vi "simflight.vi"() -> ()   [LabVIEW 2014]
uses:
  <vilib>/addons/Control Design/_Model Construction/Model Creation.llb/Model Creation SubVI/cd_Create State Space Model.vi
  <vilib>/addons/Control Design/_Utility/Model Viewer.llb/Model Viewer SubVI/cd_Draw State-Space Equation (SS).vi
  <vilib>/Utility/inputDevices.llb/joystickAcquire.vi
  <vilib>/addons/Control Design/_Time Response Analysis/Time Response.llb/Time Response subVI/cd_Linear Simulation (State-Space).vi
  <vilib>/addons/Control Design/_Time Response Analysis/NI_CD_Time Response.lvlib
  <vilib>/addons/Control Design/_Utility/NI_CD_Model Viewer.lvlib
  <vilib>/Analysis/NI_AALPro.lvlib
  <vilib>/Analysis/8numeric.llb/1D Numeric Integration.vi
  <vilib>/addons/Control Design/_Model Construction/NI_LinSys_Model Creation.lvlib
panel:
  out "flight path angle 2":dbl[](graph)
  out "XY Graph 2":cluster{"Y":dbl[], "Y":dbl[]}[](graph)
  out "horsepower":dbl[](graph)
  out "airspeed":dbl[](graph)
  out "elevator command":dbl[](graph)
  out "altitude":dbl[](graph)
  out "flight path angle":dbl[](graph)
  out "pitch rate":dbl[](graph)
  out "Equation 2":picture
  in  "stop":bool
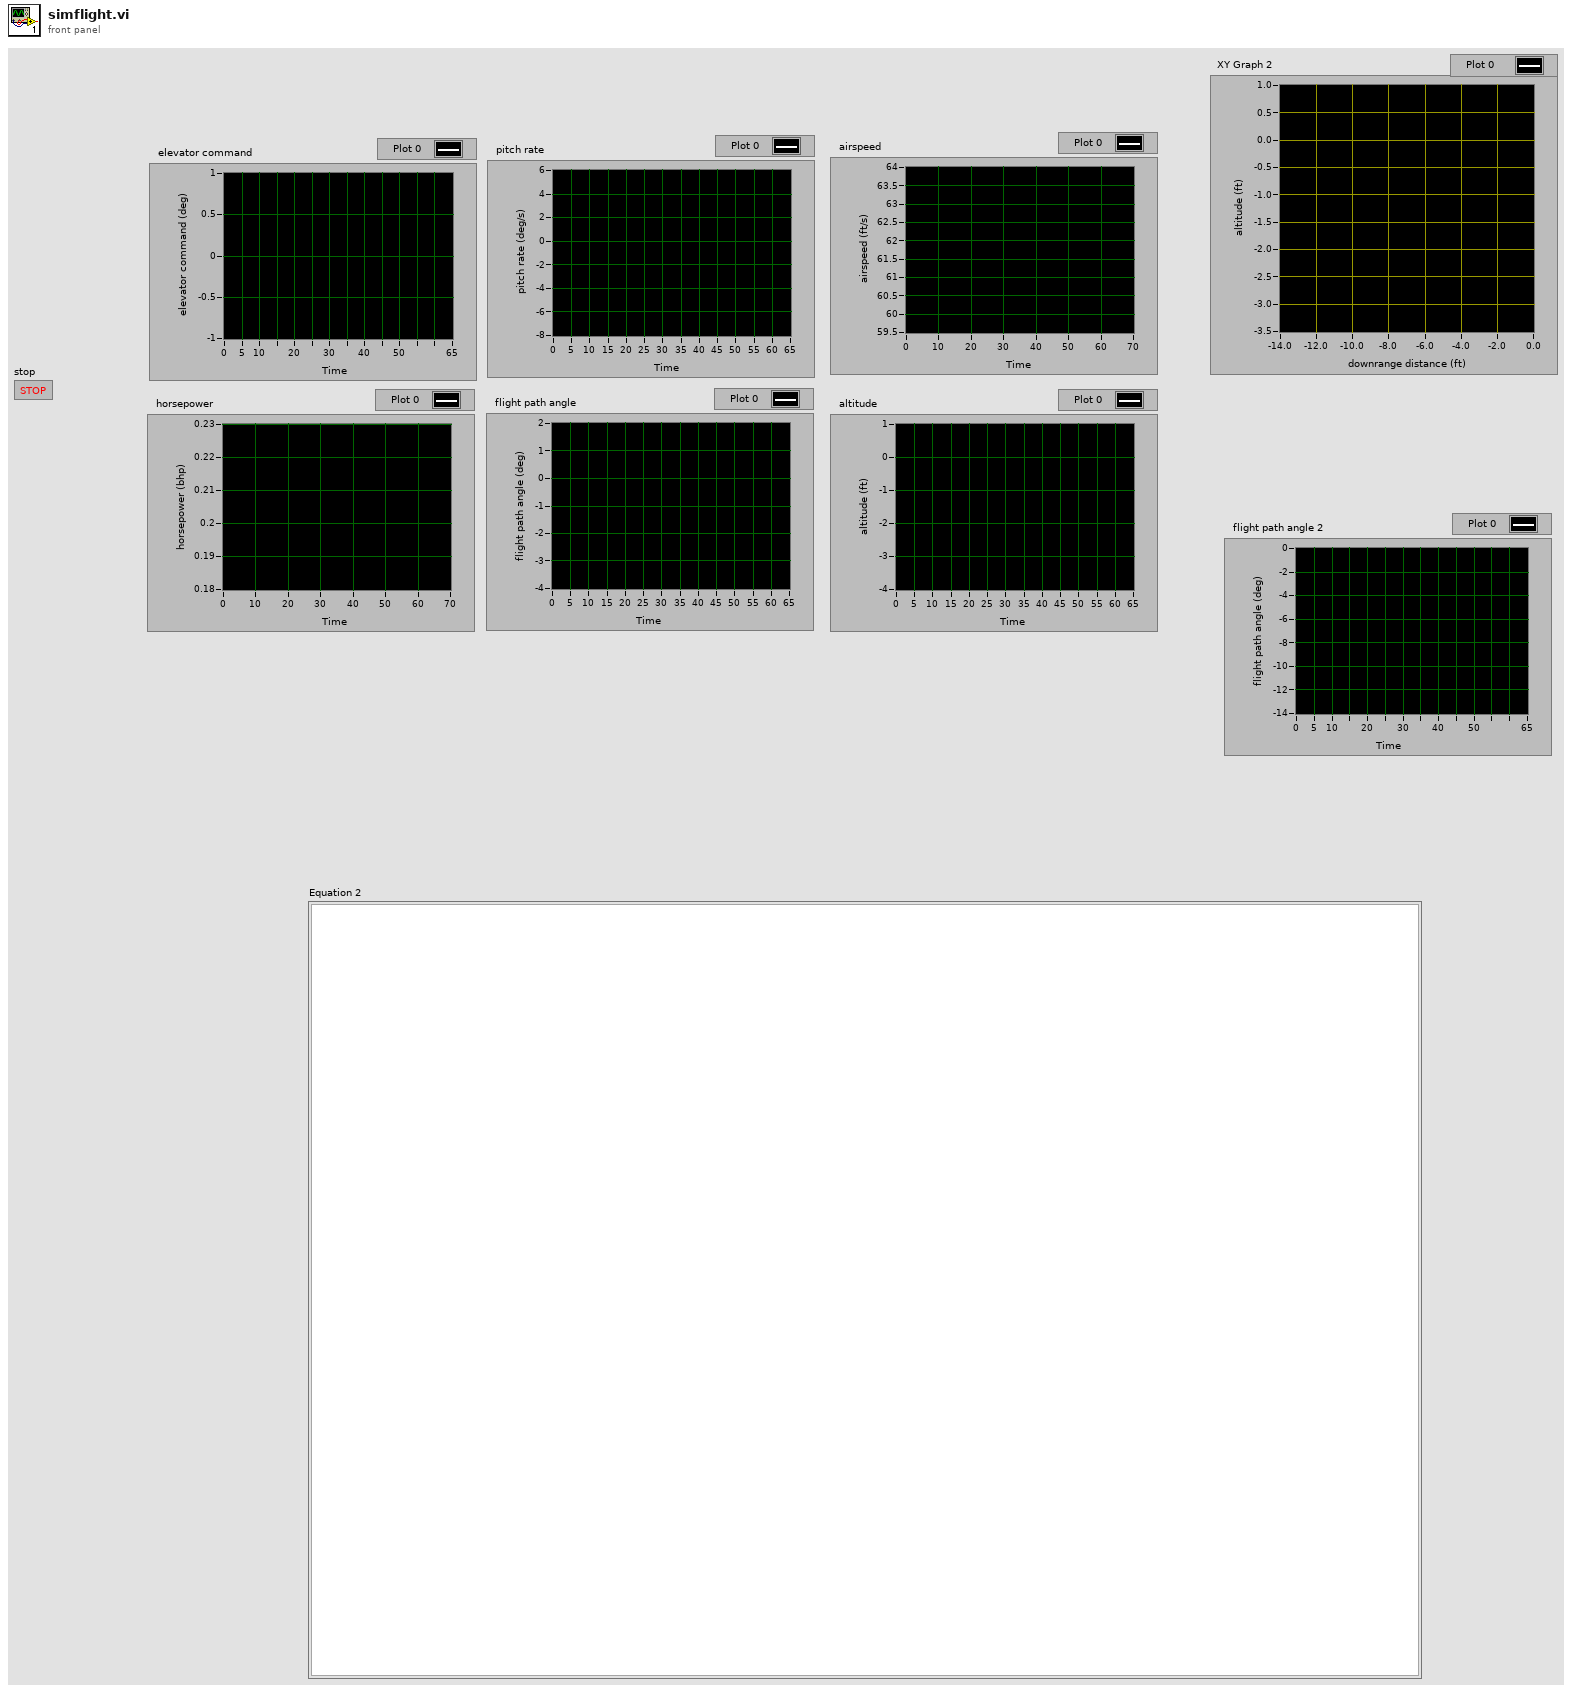
[diagram p1: front panel]
types:
  T1 = typedef "NI_LinSys_Model Typedefs.lvlib/CD State Space Model (MIMO).ctl" = cluster{"properties":T2, "A":dbl[][], "B":dbl[][], "C":dbl[][], "D":dbl[][], "StateNames":string[], "Transport Delay":dbl[][]}
  T2 = typedef "NI_LinSys_Model Typedefs.lvlib/CD General Elements.ctl" = cluster{"Model name":string, "Input names":string[], "Output names":string[], "Input Delays":dbl[], "Output Delays":dbl[], "Sampling Time":dbl, "Notes":string}
  T3 = cluster{"X axis":i32, "Y axis":i32, "Z axis":i32, "X axis rotation":i32, "Y axis rotation":i32, "Z axis rotation":i32, "U axis":i32, "V axis":i32}
  T4 = typedef "NI_LinSys_Data Typedefs.lvlib/CD MIMO Time Response Data.ctl" = cluster{"Time":dbl[], "Outputs Data":dbl[][][], "States Data":dbl[][][], "plot type":T5}
  T5 = typedef "NI_LinSys_Data Typedefs.lvlib/CD Plot Types Enum.ctl" = enum16{"bode-magnitude", "bode-phase", "nichols", "nyquist", "singular values", "step", "impulse", "initial", "simulation", "nyquist with separation"}
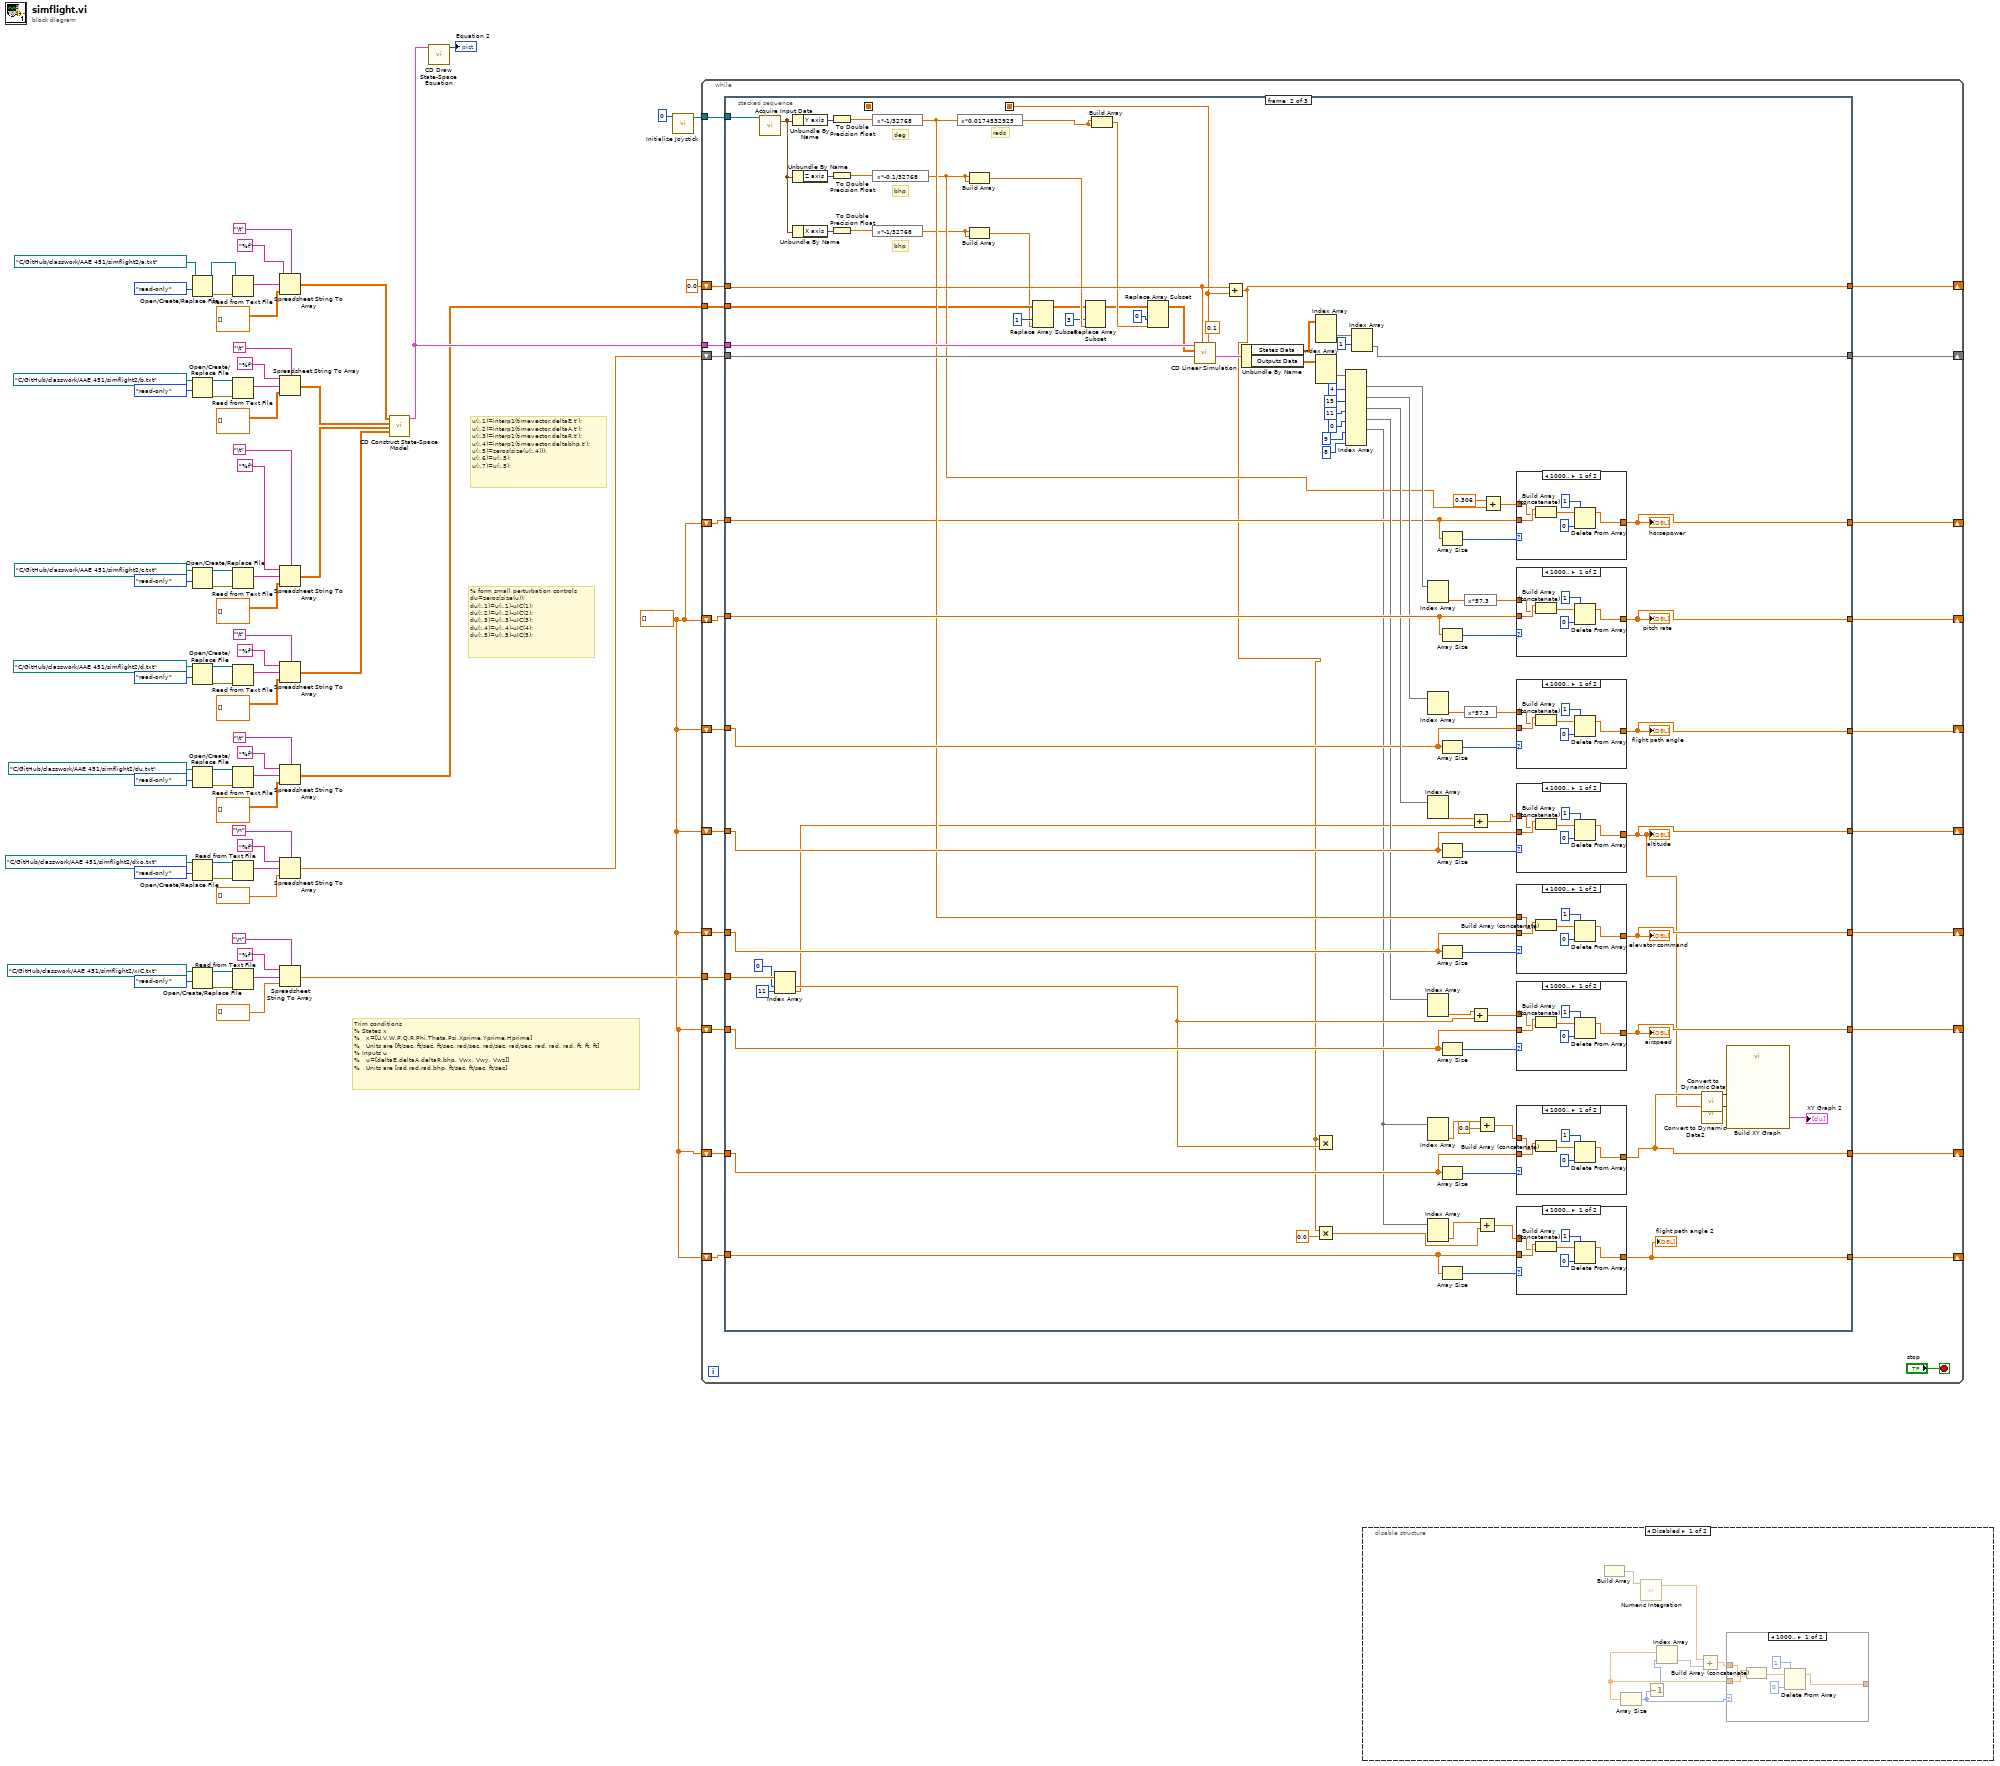
[diagram p0: block diagram]
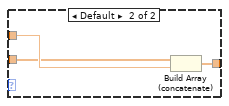
[diagram p2: hidden frame]
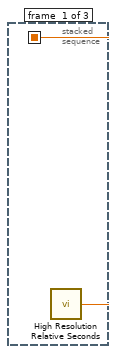
[diagram p4: hidden frame]
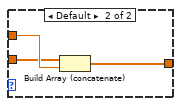
[diagram p5: hidden frame]
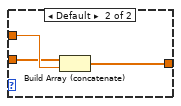
[diagram p6: hidden frame]
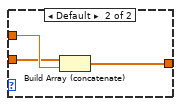
[diagram p7: hidden frame]
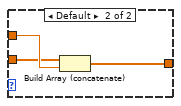
[diagram p8: hidden frame]
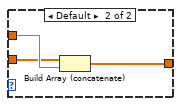
[diagram p9: hidden frame]
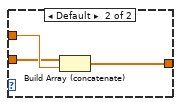
[diagram p10: hidden frame]
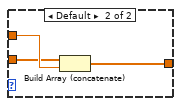
[diagram p11: hidden frame]
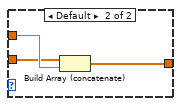
[diagram p12: hidden frame]
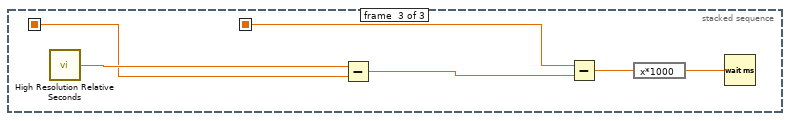
[diagram p13: hidden frame]
diagram:
  w1 = dbl[] []
  # "Trim conditions\n% States x\n%   x=[U,V,W,P,Q,R,Phi,Theta,Psi,Xprime,Yprime,Hprime]\n%   Units are [ft/sec, ft/sec, ft/sec, rad/sec, rad/sec, rad/sec, rad, rad, rad, ft, ft, ft]\n% Inputs u\n%   u=[deltaE,deltaA,deltaR,bhp, Vwx, Vwy, Vwz]]\n%   Units are [rad,rad,rad,bhp, ft/sec, ft/sec, ft/sec]"
  # "% form small perturbation controls\ndu=zeros(size(u));\ndu(:,1)=u(:,1)-uIC(1);\ndu(:,2)=u(:,2)-uIC(2);\ndu(:,3)=u(:,3)-uIC(3);\ndu(:,4)=u(:,4)-uIC(4);\ndu(:,5)=u(:,5)-uIC(5);"
  # "u(:,1)=interp1(timevector,deltaE,t');\nu(:,2)=interp1(timevector,deltaA,t');\nu(:,3)=interp1(timevector,deltaR,t');\nu(:,4)=interp1(timevector,deltabhp,t');\nu(:,5)=zeros(size(u(:,4)));\nu(:,6)=u(:,5);\nu(:,7)=u(:,5);"
  n1 = Open/Create/Replace File(file path (use dialog)=path "C:/GitHub/classwork/AAE 451/simflight2/a.txt", access (0:read/write)=enum16{"read/write", "read-only", "write-only"}."read-only") -> (refnum out=w62:refnum<file>, error out=w63:errorcluster)  [unwired: 4 in, 1 out]
  n2 = Open/Create/Replace File(file path (use dialog)=path "C:/GitHub/classwork/AAE 451/simflight2/b.txt", access (0:read/write)=enum16{"read/write", "read-only", "write-only"}."read-only") -> (refnum out=w53:refnum<file>, error out=w52:errorcluster)  [unwired: 4 in, 1 out]
  n3 = Open/Create/Replace File(file path (use dialog)=path "C:/GitHub/classwork/AAE 451/simflight2/c.txt", access (0:read/write)=enum16{"read/write", "read-only", "write-only"}."read-only") -> (refnum out=w46:refnum<file>, error out=w47:errorcluster)  [unwired: 4 in, 1 out]
  n4 = Open/Create/Replace File(file path (use dialog)=path "C:/GitHub/classwork/AAE 451/simflight2/d.txt", access (0:read/write)=enum16{"read/write", "read-only", "write-only"}."read-only") -> (refnum out=w37:refnum<file>, error out=w36:errorcluster)  [unwired: 4 in, 1 out]
  n5 = Open/Create/Replace File(file path (use dialog)=path "C:/GitHub/classwork/AAE 451/simflight2/du.txt", access (0:read/write)=enum16{"read/write", "read-only", "write-only"}."read-only") -> (refnum out=w25:refnum<file>, error out=w26:errorcluster)  [unwired: 4 in, 1 out]
  n6 = Open/Create/Replace File(file path (use dialog)=path "C:/GitHub/classwork/AAE 451/simflight2/dxo.txt", access (0:read/write)=enum16{"read/write", "read-only", "write-only"}."read-only") -> (refnum out=w15:refnum<file>, error out=w14:errorcluster)  [unwired: 4 in, 1 out]
  n7 = Open/Create/Replace File(file path (use dialog)=path "C:/GitHub/classwork/AAE 451/simflight2/xIC.txt", access (0:read/write)=enum16{"read/write", "read-only", "write-only"}."read-only") -> (refnum out=w7:refnum<file>, error out=w8:errorcluster)  [unwired: 4 in, 1 out]
  n8 = Read from Text File(file (use dialog)=w62, error in=w63) -> (text=w61:string)  [unwired: 2 in, 3 out]
  n9 = Read from Text File(file (use dialog)=w53, error in=w52) -> (text=w54:string)  [unwired: 2 in, 3 out]
  n10 = Read from Text File(file (use dialog)=w46, error in=w47) -> (text=w45:string)  [unwired: 2 in, 3 out]
  n11 = Read from Text File(file (use dialog)=w37, error in=w36) -> (text=w38:string)  [unwired: 2 in, 3 out]
  n12 = Read from Text File(file (use dialog)=w25, error in=w26) -> (text=w24:string)  [unwired: 2 in, 3 out]
  n13 = Read from Text File(file (use dialog)=w15, error in=w14) -> (text=w16:string)  [unwired: 2 in, 3 out]
  n14 = Read from Text File(file (use dialog)=w7, error in=w8) -> (text=w6:string)  [unwired: 2 in, 3 out]
  n15 = Spreadsheet String To Array(delimiter (Tab)="\t", format string="%f", spreadsheet string=w61, array type (2D Dbl)=dbl[][] []) -> (array=w33:dbl[][])
  n16 = Spreadsheet String To Array(delimiter (Tab)="\t", format string="%f", spreadsheet string=w54, array type (2D Dbl)=dbl[][] []) -> (array=w32:dbl[][])
  n17 = Spreadsheet String To Array(delimiter (Tab)="\t", format string="%f", spreadsheet string=w45, array type (2D Dbl)=dbl[][] []) -> (array=w30:dbl[][])
  n18 = Spreadsheet String To Array(delimiter (Tab)="\t", format string="%f", spreadsheet string=w38, array type (2D Dbl)=dbl[][] []) -> (array=w31:dbl[][])
  n19 = Spreadsheet String To Array(delimiter (Tab)="\t", format string="%f", spreadsheet string=w24, array type (2D Dbl)=dbl[][] []) -> (array=w20:dbl[][])
  n20 = Spreadsheet String To Array(delimiter (Tab)="\n", format string="%f", spreadsheet string=w16, array type (2D Dbl)=dbl[] []) -> (array=w11:dbl[])
  n21 = Spreadsheet String To Array(delimiter (Tab)="\n", format string="%f", spreadsheet string=w6, array type (2D Dbl)=dbl[] []) -> (array=w2:dbl[])
  n22 = call-poly <vilib>:"CD Construct State-Space Model.vi"("A"=w33, "B"=w32, "C"=w30, "D"=w31) -> ("State-Space Model"=w29:T1)  [unwired: 10 in, 1 out]
  n23 = call-poly <vilib>:"CD Draw State-Space Equation.vi"("State-Space Model"=w29) -> ("Equation"=→"Equation 2":picture)  [unwired: 8 in, 2 out]
  n24 = call <vilib>:"Initialize Joystick.vi"("device index"=0) -> ("device ID"=w66:refnum<k1>)  [unwired: 9 in, 1 out]
  n25 = while {
    shift-right: [w89] -> _
    shift-left: w11 -> [w90]
    tunnel: w29 -> [w94]
    shift-right: [w91] -> _
    shift-left: 0.0 ("Numeric") -> [w92]
    shift-right: [w87] -> _
    shift-left: w1 -> [w86]
    tunnel: w66 -> [w88]
    tunnel: w20 -> [w85]
    shift-right: [w84] -> _
    shift-left: w1 -> [w82]
    shift-right: [w83] -> _
    shift-left: w1 -> [w81]
    shift-right: [w79] -> _
    shift-left: w1 -> [w80]
    shift-right: [w77] -> _
    shift-left: w1 -> [w78]
    shift-right: [w76] -> _
    shift-left: w1 -> [w75]
    tunnel: w2 -> [w74]
    shift-right: [w72] -> _
    shift-left: w1 -> [w73]
    shift-right: [w71] -> _
    shift-left: w1 -> [w70]
    stop <- "stop" stop-if-true
    n26 = stacked-sequence {
      seq-local: [_ w161 _] -> [_ _ w265]
      seq-local: [w95 _ _] -> [_ _ w266]
      tunnel: w94 -> [_ w189 _]
      tunnel: w92 -> [_ w188 _]
      tunnel: [_ w100 _] -> w91
      tunnel: w90 -> [_ w187 _]
      tunnel: [_ w180 _] -> w89
      tunnel: w88 -> [_ w179 _]
      tunnel: [_ w178 _] -> w87
      tunnel: w86 -> [_ w177 _]
      tunnel: w85 -> [_ w109 _]
      tunnel: [_ w164 _] -> w84
      tunnel: [_ w116 _] -> w83
      tunnel: w82 -> [_ w163 _]
      tunnel: w81 -> [_ w162 _]
      tunnel: [_ w159 _] -> w79
      tunnel: w80 -> [_ w160 _]
      tunnel: [_ w148 _] -> w77
      tunnel: w78 -> [_ w147 _]
      tunnel: [_ w118 _] -> w76
      tunnel: w75 -> [_ w144 _]
      tunnel: w74 -> [_ w141 _]
      tunnel: [_ w126 _] -> w72
      tunnel: w73 -> [_ w127 _]
      tunnel: [_ w97 _] -> w71
      tunnel: w70 -> [_ w101 _]
      frame #0 {
        n27 = call <vilib>:"High Resolution Relative Seconds.vi"() -> ("relative seconds"=w95:dbl)
      }
      frame #1 {
        w161 = 0.1 ("Delta t")
        # "bhp"
        # "bhp"
        # "rads"
        # "deg"
        n28 = call-poly <vilib>:"Acquire Input Data.vi"("device ID"=w179) -> ("axis info"=w111:T3)  [unwired: 14 in, 4 out]
        n29 = Index Array(array=w141, index #1=0 ("index"), index #2=11 ("index")) -> (element #1=w138:dbl, element #2=w131:dbl)
        n30 = Unbundle By Name(w111) -> ("Y axis"=w155:i32)
        n31 = Unbundle By Name(w111) -> ("Z axis"=w129:i32)
        n32 = Unbundle By Name(w111) -> ("X axis"=w113:i32)
        n33 = To Double Precision Float(number=w155) -> (double precision float=w154:dbl)
        n34 = To Double Precision Float(number=w129) -> (double precision float=w130:dbl)
        n35 = To Double Precision Float(number=w113) -> (double precision float=w112:dbl)
        n36 = expression code="x*-1/32768"(w154) -> (w153:dbl)
        n37 = expression code="x*-0.1/32768"(w130) -> (w121:dbl)
        n38 = expression code="x*-1/32768"(w112) -> (w114:dbl)
        n39 = expression code="x*0.0174532925"(w153) -> (w152:dbl)
        n40 = Build Array(w121, w121) -> (w124:dbl[])
        n41 = Build Array(w114, w114) -> (w107:dbl[])
        n42 = Replace Array Subset(array=w109, new element=w107, index (col)=1 ("disabled index (col)")) -> (w108:dbl[][])  [unwired: 1 in]
        n43 = Replace Array Subset(array=w108, new element=w124, index (col)=3 ("disabled index (col)")) -> (w125:dbl[][])  [unwired: 1 in]
        n44 = Build Array(w152, w152) -> (w175:dbl[])
        n45 = Replace Array Subset(array=w125, new element=w175, index (col)=0 ("index")) -> (w173:dbl[][])  [unwired: 1 in]
        n46 = call-poly <vilib>:"CD Linear Simulation.vi"("Delta t"=w161, "Initial Time"=w188, "Initial Conditions"=w187, "Inputs"=w173, "State-Space Model"=w189) -> ("Simulation Data"=w183:T4)  [unwired: 3 in, 3 out]
        n47 = Add(x=w188, y=w161) -> (x+y=w100:dbl)
        n48 = Unbundle By Name(w183) -> ("States Data"=w171:dbl[][][], "Outputs Data"=w172:dbl[][][])
        n49 = Index Array(array=w171) -> (element=w182:dbl[][])  [unwired: 3 in]
        n50 = Index Array(array=w172) -> (element=w186:dbl[][])  [unwired: 3 in]
        n51 = Multiply(x=w100, y=w138) -> ()  [unwired: 1 out]
        n52 = Multiply(x=w100, y=0.0) -> (x*y=w98:dbl)
        n53 = Index Array(array=w186, index (col) #1=4 ("disabled index (col)"), index (col) #2=15 ("disabled index (col)"), index (col) #3=11 ("disabled index (col)"), index (col) #4=0 ("disabled index (col)"), index (col) #5=9 ("index (col)"), index (col) #6=8 ("index (col)")) -> (element #1=w184:dbl[], element #2=w166:dbl[], element #3=w165:dbl[], element #4=w145:dbl[], element #5=w102:dbl[])  [unwired: 6 in, 1 out]
        n54 = Index Array(array=w182, index (row)=1) -> (element=w180:dbl[])  [unwired: 1 in]
        n55 = Index Array(array=w184) -> (element #2=w157:dbl)  [unwired: 2 in, 1 out]
        n56 = Index Array(array=w166) -> (element #2=w151:dbl)  [unwired: 2 in, 1 out]
        n57 = Index Array(array=w165) -> (element #2=w134:dbl)  [unwired: 2 in, 1 out]
        n58 = Index Array(array=w145) -> (element #2=w140:dbl)  [unwired: 2 in, 1 out]
        n59 = Index Array(array=w102) -> (element #2=w137:dbl)  [unwired: 2 in, 1 out]
        n60 = Index Array(array=w102) -> (element #2=w104:dbl)  [unwired: 2 in, 1 out]
        n61 = Array Size(array=w127) -> (size(s)=w128:i32)
        n62 = Array Size(array=w177) -> (size(s)=w176:i32)
        n63 = Array Size(array=w163) -> (size(s)=w168:i32)
        n64 = Array Size(array=w162) -> (size(s)=w167:i32)
        n65 = Array Size(array=w160) -> (size(s)=w158:i32)
        n66 = Array Size(array=w147) -> (size(s)=w149:i32)
        n67 = Array Size(array=w144) -> (size(s)=w143:i32)
        n68 = Array Size(array=w101) -> (size(s)=w103:i32)
        n69 = expression code="x*57.3"(w157) -> (w156:dbl)
        n70 = expression code="x*57.3"(w151) -> (w150:dbl)
        n71 = Add(x=w134, y=w131) -> (x+y=w135:dbl)
        n72 = Add(x=w140, y=w138) -> (x+y=w139:dbl)
        n73 = Add(x=w137, y=0.0) -> (x+y=w136:dbl)
        n74 = Add(x=w104, y=w98) -> (x+y=w105:dbl)
        n75 = Add(x=0.306, y=w121) -> (x+y=w122:dbl)
        n76 = case shown="1000.." w128 {
          tunnel: w122 -> [w203 w207]
          tunnel: [w199 w206] -> w126
          tunnel: w127 -> [w204 w205]
          frame 1000.. {
            n77 = Build Array (concatenate)(w204, w203) -> (w202:dbl[])
            n78 = Delete From Array(array=w202, length=1, index=0) -> (array with subset deleted=w199:dbl[])  [unwired: 1 out]
          }
          frame Default {
            n79 = Build Array (concatenate)(w205, w207) -> (w206:dbl[])
          }
        }
        "horsepower" <- w126
        n80 = case shown="1000.." w176 {
          tunnel: w156 -> [w257 w261]
          tunnel: [w253 w260] -> w178
          tunnel: w177 -> [w258 w259]
          frame 1000.. {
            n81 = Build Array (concatenate)(w258, w257) -> (w256:dbl[])
            n82 = Delete From Array(array=w256, length=1, index=0) -> (array with subset deleted=w253:dbl[])  [unwired: 1 out]
          }
          frame Default {
            n83 = Build Array (concatenate)(w259, w261) -> (w260:dbl[])
          }
        }
        "pitch rate" <- w178
        n84 = case shown="1000.." w168 {
          tunnel: w150 -> [w248 w252]
          tunnel: [w244 w251] -> w164
          tunnel: w163 -> [w249 w250]
          frame 1000.. {
            n85 = Build Array (concatenate)(w249, w248) -> (w247:dbl[])
            n86 = Delete From Array(array=w247, length=1, index=0) -> (array with subset deleted=w244:dbl[])  [unwired: 1 out]
          }
          frame Default {
            n87 = Build Array (concatenate)(w250, w252) -> (w251:dbl[])
          }
        }
        "flight path angle" <- w164
        n88 = case shown="1000.." w167 {
          tunnel: w135 -> [w239 w243]
          tunnel: [w235 w242] -> w116
          tunnel: w162 -> [w240 w241]
          frame 1000.. {
            n89 = Build Array (concatenate)(w240, w239) -> (w238:dbl[])
            n90 = Delete From Array(array=w238, length=1, index=0) -> (array with subset deleted=w235:dbl[])  [unwired: 1 out]
          }
          frame Default {
            n91 = Build Array (concatenate)(w241, w243) -> (w242:dbl[])
          }
        }
        "altitude" <- w116
        n92 = case shown="1000.." w158 {
          tunnel: w153 -> [w230 w234]
          tunnel: [w226 w233] -> w159
          tunnel: w160 -> [w231 w232]
          frame 1000.. {
            n93 = Build Array (concatenate)(w231, w230) -> (w229:dbl[])
            n94 = Delete From Array(array=w229, length=1, index=0) -> (array with subset deleted=w226:dbl[])  [unwired: 1 out]
          }
          frame Default {
            n95 = Build Array (concatenate)(w232, w234) -> (w233:dbl[])
          }
        }
        "elevator command" <- w159
        n96 = case shown="1000.." w149 {
          tunnel: w139 -> [w221 w225]
          tunnel: [w217 w224] -> w148
          tunnel: w147 -> [w222 w223]
          frame 1000.. {
            n97 = Build Array (concatenate)(w222, w221) -> (w220:dbl[])
            n98 = Delete From Array(array=w220, length=1, index=0) -> (array with subset deleted=w217:dbl[])  [unwired: 1 out]
          }
          frame Default {
            n99 = Build Array (concatenate)(w223, w225) -> (w224:dbl[])
          }
        }
        "airspeed" <- w148
        n100 = case shown="1000.." w143 {
          tunnel: w136 -> [w212 w216]
          tunnel: [w208 w215] -> w118
          tunnel: w144 -> [w213 w214]
          frame 1000.. {
            n101 = Build Array (concatenate)(w213, w212) -> (w211:dbl[])
            n102 = Delete From Array(array=w211, length=1, index=0) -> (array with subset deleted=w208:dbl[])  [unwired: 1 out]
          }
          frame Default {
            n103 = Build Array (concatenate)(w214, w216) -> (w215:dbl[])
          }
        }
        n104 = case shown="1000.." w103 {
          tunnel: w105 -> [w194 w198]
          tunnel: [w190 w197] -> w97
          tunnel: w101 -> [w195 w196]
          frame 1000.. {
            n105 = Build Array (concatenate)(w195, w194) -> (w193:dbl[])
            n106 = Delete From Array(array=w193, length=1, index=0) -> (array with subset deleted=w190:dbl[])  [unwired: 1 out]
          }
          frame Default {
            n107 = Build Array (concatenate)(w196, w198) -> (w197:dbl[])
          }
        }
        "flight path angle 2" <- w97
        n108 = call "Convert to Dynamic Data"("Array"=w118) -> ("Dynamic Data Type"=w117:dynamicdata)  [unwired: 3 in]
        n109 = call "Convert to Dynamic Data2"("Array"=w116) -> ("Dynamic Data Type"=w115:dynamicdata)  [unwired: 3 in]
        n110 = call "Build XY Graph"("Y Input"=w115, "X Input"=w117) -> ("XY Graph"=→"XY Graph 2":cluster{"X":dbl[], "Y":dbl[]}[])  [unwired: 8 in, 1 out]
      }
      frame #2 {
        n111 = call <vilib>:"High Resolution Relative Seconds.vi"() -> ("relative seconds"=w267:dbl)
        n112 = Subtract(x=w267, y=w266) -> (x-y=w264:dbl)
        n113 = Subtract(x=w265, y=w264) -> (x-y=w263:dbl)
        n114 = expression code="x*1000"(w263) -> (w262:dbl)
        n115 = Wait (ms)(milliseconds to wait=w262) -> ()  [unwired: 1 out]
      }
    }
  }
  n116 = disable-structure shown="Disabled" {
    frame Disabled {
      n117 = Build Array() -> (w268:void[])  [unwired: 2 in]
      n118 = call-poly <vilib>:"Numeric Integration.vi"("Input Array"=w268) -> ("result"=w270:dbl, "dt"=w275:dbl)  [unwired: 1 in, 1 out]
      n119 = Array Size(array=w269) -> (size(s)=w271:i32)
      n120 = Decrement(x=w271) -> (x-1=w272:i32)
      n121 = Index Array(array=w269, index=w272) -> (element=w273)
      n122 = Add(x=w270, y=w273) -> (x+y=w274:dbl)
      n123 = case shown="1000.." w271 {
        tunnel: w274 -> [w280 w284]
        tunnel: [w276 w283] -> _
        tunnel: [w281 w282] -> w269
        frame 1000.. {
          n124 = Build Array (concatenate)(w281, w280) -> (w279:dbl[])
          n125 = Delete From Array(array=w279, length=1, index=0) -> (array with subset deleted=w276:dbl[])  [unwired: 1 out]
        }
        frame Default {
          n126 = Build Array (concatenate)(w282, w284) -> (w283:dbl[])
        }
      }
    }
    frame Enabled {
    }
  }
